vi "AdjustPreflashTimings.vi"(1 "Input Trigger Data":T3) -> (0 "Output Trigger Data":T3)   [LabVIEW 2016]
uses:
  Ctrl_Signal.ctl
  Ctrl_Signal_Map.ctl
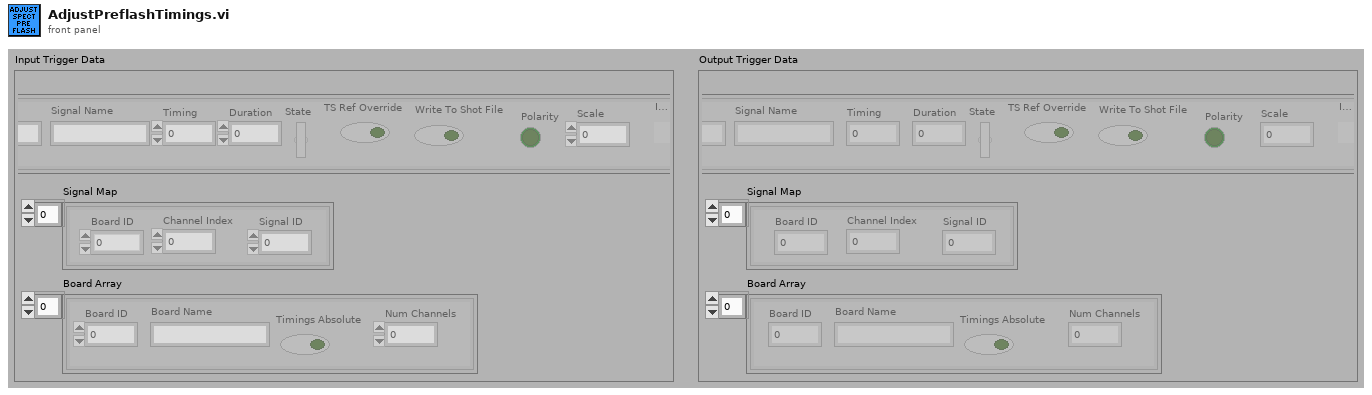
[diagram p1: front panel]
types:
  T1 = typedef "Ctrl_Signal.ctl" = cluster{"Signal Name":string, "Timing":dbl, "Duration":dbl, "State":bool, "TS Ref Override":bool, "Write To Shot File":bool, "Polarity":bool, "Signal ID":dbl, "Scale":dbl, "IsDelay":bool}
  T2 = typedef "Ctrl_Signal_Map.ctl" = cluster{"Channel Index":dbl, "Board ID":dbl, "Signal ID":dbl}
  T3 = cluster{"Signal Array":T1[], "Signal Map":T2[], "Board Array":cluster{"Board ID":dbl, "Board Name":string, "Timings Absolute":bool, "Num Channels":dbl}[]}
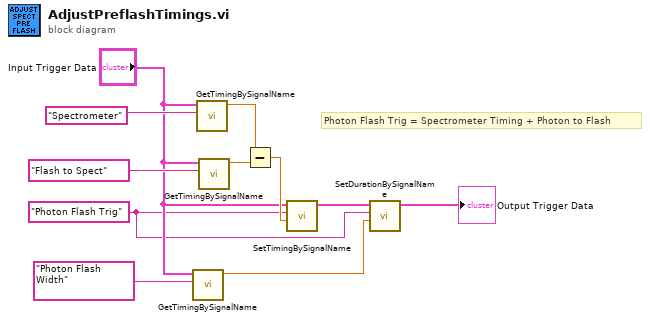
[diagram p0: block diagram]
diagram:
  w2 = "Photon Flash Trig" ("Signal Name")
  # "Photon Flash Trig = Spectrometer Timing + Photon to Flash"
  n1 = call "GetTimingBySignalName.vi"("Signal Name"="Photon Flash Width", "Trigger Data"="Input Trigger Data") -> ("Timing"=w3:dbl)  [unwired: 9 in]
  n2 = call "GetTimingBySignalName.vi"("Signal Name"="Spectrometer", "Trigger Data"="Input Trigger Data") -> ("Timing"=w9:dbl)  [unwired: 9 in]
  n3 = call "GetTimingBySignalName.vi"("Signal Name"="Flash to Spect", "Trigger Data"="Input Trigger Data") -> ("Timing"=w8:dbl)  [unwired: 9 in]
  n4 = Subtract(x=w9, y=w8) -> (x-y=w7:dbl)
  n5 = call "SetTimingBySignalName.vi"("Timing"=w7, "Signal Name"=w2, "Trigger Data Input"="Input Trigger Data") -> ("Trigger Data Output"=w1:T3)  [unwired: 8 in]
  n6 = call "SetDurationBySignalName.vi"("Duration"=w3, "Signal Name"=w2, "Trigger Data Input"=w1) -> ("Trigger Data Output"=→"Output Trigger Data":T3)  [unwired: 8 in]
